vi "Generator High Speed PIDDW.vi"() -> ()   [LabVIEW 2024]
uses:
  <vilib>/Instr/_visa.llb/VISA Configure Serial Port (Instr).vi
panel:
  in  "ReInit":bool
  in  "Output Limits":cluster{"Hi":dbl, "Low":dbl}={"Hi"=255.0, "Low"=-255.0}
  in  "PID Coefficients":cluster{"P":dbl, "I":dbl, "D":dbl}={"P"=2.0, "I"=5.0, "D"=0.0}
  out "Output":u8=132
  out "Error":i16=-15
  out "mWatts":sgl=30.482622 format="%#_3g"
  out "Freq. Hz":dbl=48.78048780487805 format="%#_3g"
  out "dt out (s)":dbl=0.0205 format="%.3f"
  in  "Loop Per":dbl(slide)=1.0 scale=0.0..50.0
  in  "V Setpoint":i16(slide)=582 scale=0.0..1000.0
  in  "Load Level":u8(slide)=88 scale=0.0..255.0
  in  "stop":bool
  out "Waveform Chart":cluster{"V Setpoint":i16, i16}(graph)={"V Setpoint"=582, 597}
  in  "baud rate (9600)":u32=115200
  in  "VISA resource name":refnum<visa-resource-name>="COM28"
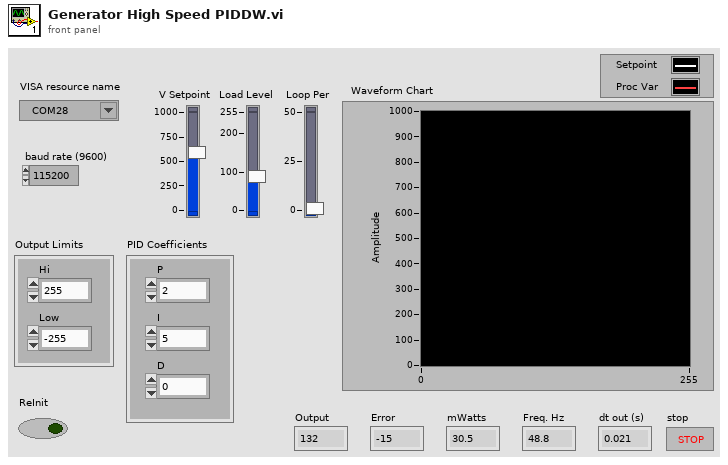
[diagram p1: front panel]
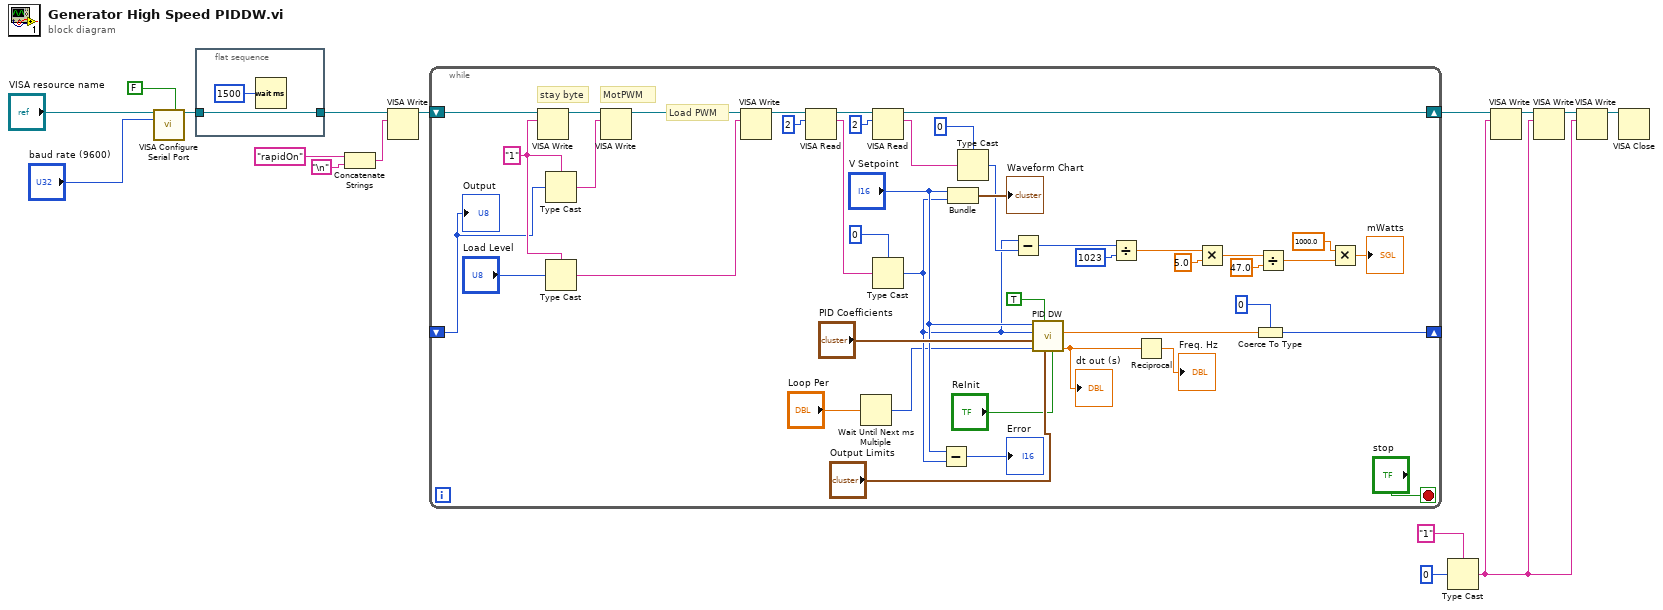
[diagram p0: block diagram]
diagram:
  n1 = call-poly "VISA Configure Serial Port"("VISA resource name"="VISA resource name", "Enable Termination\nChar (T)"=FALSE ("Enable Termination\nChar (T)"), "baud rate (9600)"="baud rate (9600)") -> ("VISA resource name out"=w11:refnum<visa-resource-name>)  [unwired: 11 in, 1 out]
  n2 = flat-sequence {
    tunnel: w11 -> [w17]
    tunnel: [w17] -> w10
    frame #0 {
      n3 = Wait (ms)(milliseconds to wait=u32 1500) -> ()  [unwired: 1 out]
    }
  }
  n4 = Concatenate Strings("rapidOn" ("string"), "\n") -> (w14:string)
  n5 = VISA Write(VISA resource name=w10, write buffer=w14) -> (VISA resource name out=w9:refnum<visa-resource-name>)  [unwired: 1 in, 2 out]
  n6 = while {
    shift-right: [w43] -> w5
    shift-left: w9 -> [w61]
    shift-right: [w46] -> _
    shift-left: _ -> [w49]
    stop <- "stop" stop-if-true
    w50 = "1"
    # "Load PWM"
    # "MotPWM"
    # "stay byte"
    n7 = VISA Write(VISA resource name=w61, write buffer=w50) -> (VISA resource name out=w56:refnum<visa-resource-name>)  [unwired: 1 in, 2 out]
    n8 = Type Cast(type=w50, x=w49) -> (*(type *) &x=w53:string)
    n9 = Type Cast(type=w50, x="Load Level") -> (*(type *) &x=w51:string)
    n10 = VISA Write(VISA resource name=w56, write buffer=w53) -> (VISA resource name out=w59:refnum<visa-resource-name>)  [unwired: 1 in, 2 out]
    n11 = VISA Write(VISA resource name=w59, write buffer=w51) -> (VISA resource name out=w58:refnum<visa-resource-name>)  [unwired: 1 in, 2 out]
    n12 = VISA Read(VISA resource name=w58, byte count=u32 2) -> (VISA resource name out=w44:refnum<visa-resource-name>, read buffer=w55:string)  [unwired: 1 in, 2 out]
    n13 = Wait Until Next ms Multiple(millisecond multiple="Loop Per") -> (millisecond timer value=w19:u32)
    n14 = VISA Read(VISA resource name=w44, byte count=u32 2) -> (VISA resource name out=w43:refnum<visa-resource-name>, read buffer=w41:string)  [unwired: 1 in, 2 out]
    n15 = Type Cast(type=i16 0, x=w55) -> (*(type *) &x=w23:i16)
    n16 = Subtract(x="V Setpoint", y=w23) -> (x-y=→"Error":i16)
    n17 = Bundle("V Setpoint"="V Setpoint", w23) -> (→"Waveform Chart":cluster{"V Setpoint":i16, i16})  [unwired: 1 in]
    n18 = Type Cast(type=i16 0, x=w41) -> (*(type *) &x=w40:i16)
    n19 = Subtract(x=w23, y=w40) -> (x-y=w36:i16)
    n20 = call "PID DW.vi"("Init?"="ReInit", "Output Limits"="Output Limits", "Auto/Manual"=TRUE, "dT(in)"=w19, "PID Coefficients"="PID Coefficients", "Process Variable"=w23, "Setpoint"="V Setpoint") -> ("dT"=w20:dbl, "Output"=w29:dbl)  [unwired: 3 in]
    "dt out (s)" <- w20
    n21 = Divide(x=w36, y=i16 1023) -> (x/y=w34:dbl)
    n22 = Reciprocal(x=w20) -> (1/x=→"Freq. Hz":dbl)
    n23 = Multiply(x=w34, y=5.0) -> (x*y=w32:dbl)
    n24 = Coerce To Type(0:w29, 1:u8 0) -> (2:w46:u8)
    n25 = Divide(x=w32, y=sgl 47.0) -> (x/y=w38:dbl)
    n26 = Multiply(x=1000.0, y=w38) -> (x*y=→"mWatts":dbl)
    "Output" <- w49
  }
  n27 = Type Cast(type="1", x=u32 0 ("millisecond multiple")) -> (*(type *) &x=w3:string)
  n28 = VISA Write(VISA resource name=w5, write buffer=w3) -> (VISA resource name out=w6:refnum<visa-resource-name>)  [unwired: 1 in, 2 out]
  n29 = VISA Write(VISA resource name=w6, write buffer=w3) -> (VISA resource name out=w7:refnum<visa-resource-name>)  [unwired: 1 in, 2 out]
  n30 = VISA Write(VISA resource name=w7, write buffer=w3) -> (VISA resource name out=w4:refnum<visa-resource-name>)  [unwired: 1 in, 2 out]
  n31 = VISA Close(VISA resource name=w4) -> ()  [unwired: 1 in, 1 out]
